vi "Documentation.vi"   [LabVIEW 2018]
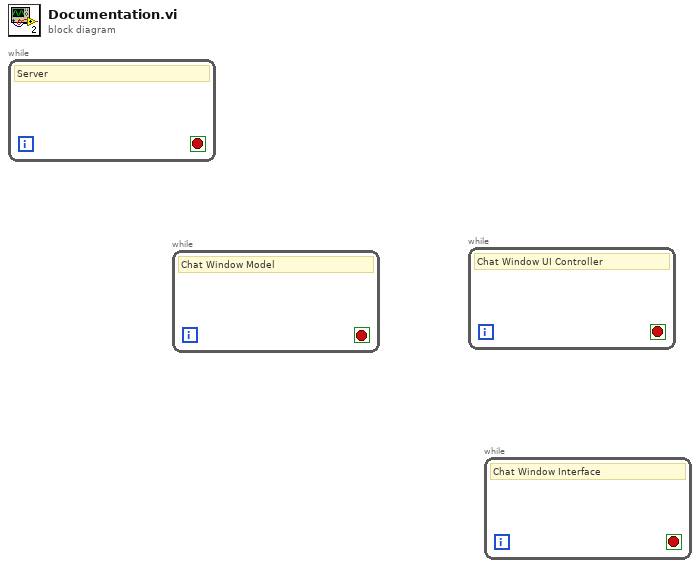
[diagram p0: block diagram]
diagram:
  n1 = while {
    stop <- _ stop-if-true
    # "Server"
  }
  n2 = while {
    stop <- _ stop-if-true
    # "Chat Window Model"
  }
  n3 = while {
    stop <- _ stop-if-true
    # "Chat Window UI Controller"
  }
  n4 = while {
    stop <- _ stop-if-true
    # "Chat Window Interface"
  }
